vi "SetSoftTrig.vi"(8 "SoftTrig":bool=TRUE, 11 "error in":errorcluster caption="错误输入") -> (3 "error out":errorcluster caption="错误输出")   [LabVIEW 2016]
uses:
  PLC-Lab/lib/gusb.dll
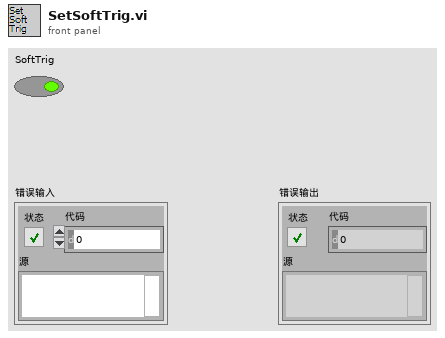
[diagram p1: front panel]
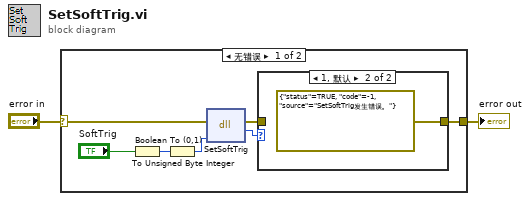
[diagram p0: block diagram]
diagram:
  n1 = case shown="无错误" "error in" {
    selector: "error in" -> [w8 w12]
    tunnel: [w9 w12] -> w1
    frame No Error {
      n2 = Boolean To (0,1)(Boolean="SoftTrig") -> (0, 1=w5:i16)
      n3 = To Unsigned Byte Integer(number=w5) -> (unsigned 8bit integer=w3:u8)
      n4 = dll-call lib="E:/Camproject/2018/2018.1Labview/PLC-Lab/lib/gusb.dll" fn="SetSoftTrig"(error in=w8, "Trig"=w3) -> (error out=w6:errorcluster, "Status"=w7:i32)  [unwired: 3 in, 1 out]
      n5 = case shown="1, 默认" w7 {
        tunnel: [w10 errorcluster {"status"=TRUE, "code"=-1, "source"="SetSoftTrig发生错误。"} ("错误常量")] -> w9
        tunnel: w6 -> [w10 _]
        frame 0 {
        }
        frame 1, Default {
        }
      }
    }
    frame Error {
    }
  }
  "error out" <- w1
